vi "Build_Plot_Selection-Playback.vi"(7 "File Info":T1, 8 "error in (no error)":errorcluster) -> (0 "error out":errorcluster, 3 "Plot Selection":T2(array[cluster]))   [LabVIEW 2020]
uses:
  <vilib>/Dataflow_G/G-Audio/Controls/Audio File Info.ctl
  <vilib>/Dataflow_G/G-Audio/G-Audio.lvlib
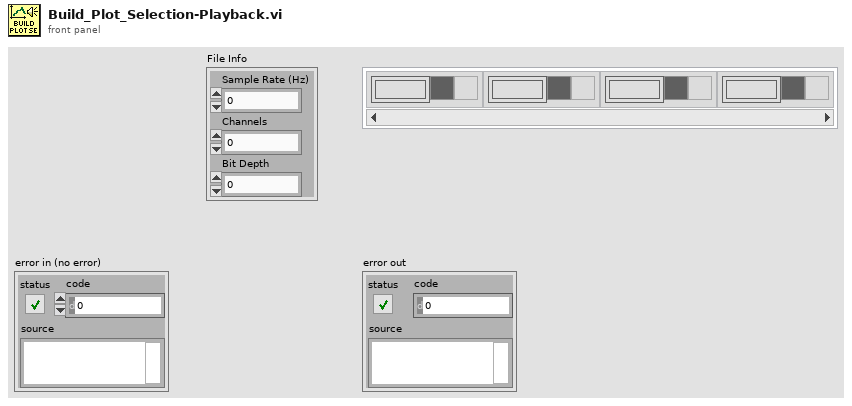
[diagram p1: front panel]
types:
  T1 = typedef "G-Audio.lvlib/Audio File Info.ctl" = cluster{"Sample Rate (Hz)":u32, "Channels":u32, "Bit Depth":u32}
  T2 = cluster{"Plot Name":string, "Plot Color":u32, "Visibility":bool}[]
  T3 = cluster{"Plot Name":string, "Plot Color":u32, "Visibility":bool}
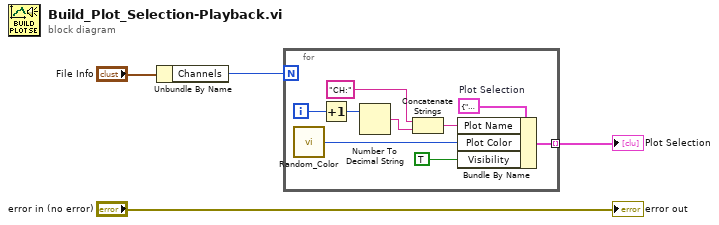
[diagram p0: block diagram]
diagram:
  n1 = Unbundle By Name("File Info") -> ("Channels"=w1:u32)
  n2 = for {
    N: w1 -> [_]
    tunnel: [w12] -> w4 mode=indexing
    i -> [w10]
    w13 = T3 {"Plot Name"="", "Plot Color"=0, "Visibility"=FALSE}  # Plot Selection
    n3 = call "Random_Color.vi"() -> ("Color"=w11:u32)
    n4 = Increment(x=w10) -> (x+1=w6:i32)
    n5 = Number To Decimal String(number=w6) -> (decimal integer string=w5:string)  [unwired: 1 in]
    n6 = Concatenate Strings("CH:", w5) -> (w8:string)
    n7 = Bundle By Name(cluster=w13, "Plot Name"=w8, "Plot Color"=w11, "Visibility"=TRUE) -> (w12:T3)
  }
  "Plot Selection" <- w4
  "error out" <- "error in (no error)"
